vi "Handling Mouse Events.vi"() -> ()   [LabVIEW 2023]
doc: "Shows how to utilize mouse events with the Event Structure to build a \"roll over\" display. A \"roll over\" display is one that changes a page element when the user \"rolls\" the mouse over an element on the page without actually clicking on it. One example of a \"roll over\" display in LabVIEW is the Context Help window, which changes its content as the mouse hovers over different items in the VI."
panel:
  in  "Empty Space Text":string="(Empty Space)"
  in  "Boolean":bool
  in  "Waveform":waveform(dbl)
  in  "Vertical Fill Slide":dbl(slide) scale=0.0..10.0
  in  "Stop":bool
  out "Mouse Over Item":string
  in  "Numeric Control":dbl
  # "Overview: Demonstrates the use of the Event Structure to handle mouse events.\nInstructions:\n1. Run the VI.\n2. Move your mouse around the front panel. As you hover over controls, their labels should appear in the Mouse Over Item display.\n3. Click Stop to stop the VI."
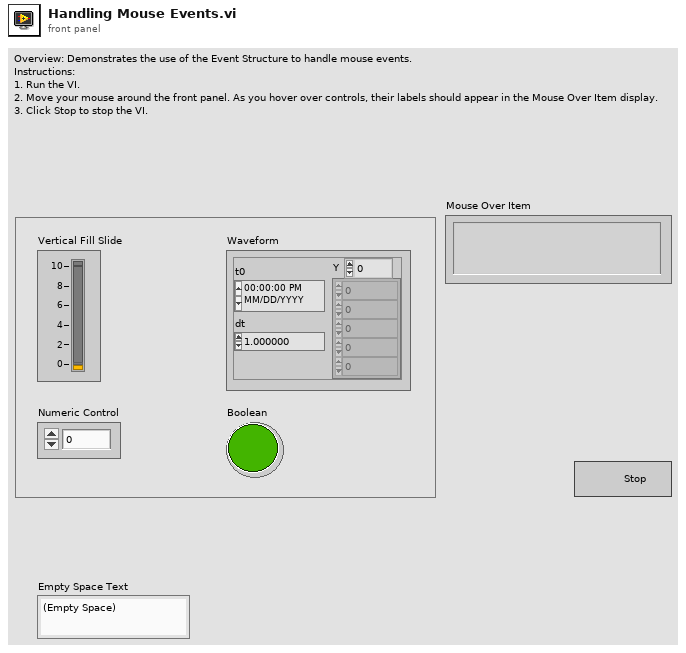
[diagram p1: front panel]
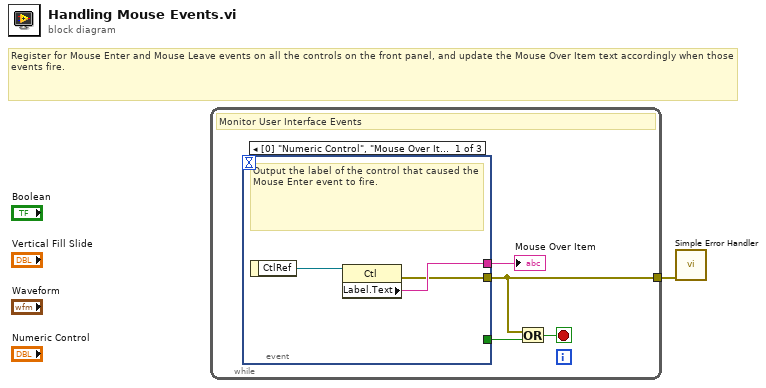
[diagram p0: block diagram]
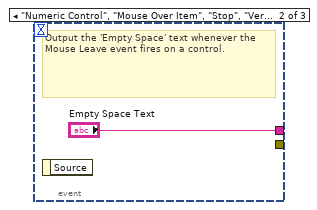
[diagram p2: hidden frame]
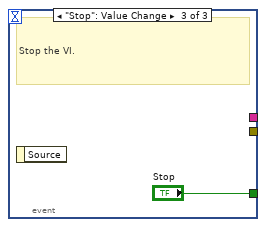
[diagram p3: hidden frame]
diagram:
  # "Register for Mouse Enter and Mouse Leave events on all the controls on the front panel, and update the Mouse Over Item text accordingly when those events fire."
  n1 = while {
    tunnel: [w2] -> w1
    stop <- w3 stop-if-true
    # "Monitor User Interface Events"
    n2 = event shown="[0] \"Numeric Control\", \"Mouse Over Item\", \"Stop\", \"Vertical Fill Slide\", \"Waveform\", \"Boolean\": Mouse Enter" {
      selector: _ -> [_ _ _]
      dyn-events: _ -> [_ _ _]
      timeout: _ -> [_ _ _]
      tunnel: [w7 "Empty Space Text" _] -> w5
      tunnel: [_ _ "Stop"] -> w4
      tunnel: [w6 _ _] -> w2
      event "Numeric Control", "Mouse Over Item", "Stop", "Vertical Fill Slide", "Waveform", "Boolean": Mouse Enter {
        # "Output the label of the control that caused the Mouse Enter event to fire."
        n3 = event-data() -> ("CtlRef"=w8:refnum<vi>)  [unwired: 1 out]
        n4 = property class="Ctl"(reference=w8) -> (error out=w6:errorcluster, "Label.Text"=w7:string)  [unwired: 1 in, 1 out]
      }
      event "Numeric Control", "Mouse Over Item", "Stop", "Vertical Fill Slide", "Waveform", "Boolean": Mouse Leave {
        # "Output the 'Empty Space' text whenever the Mouse Leave event fires on a control."
        n5 = event-data() -> ()  [unwired: 2 out]
      }
      event "Stop": Value Change {
        # "Stop the VI."
        n6 = event-data() -> ()  [unwired: 2 out]
      }
    }
    "Mouse Over Item" <- w5
    n7 = Or(x=w2, y=w4) -> (x .or. y?=w3:bool)
  }
  n8 = call <vilib>:"Simple Error Handler.vi"("error in (no error)"=w1) -> ()  [unwired: 4 in, 5 out]
